vi "Intersperse Data with Invalid Data (single channel).vi"(7 "Intersperse Ratio":dbl=0.1, 10 "Input Data":dbl[](array[numeric]) format="%.16g") -> (1 "Data Valid":bool[](array[boolean]), 2 "Output Data":dbl[](array[numeric]))   [LabVIEW 2011]
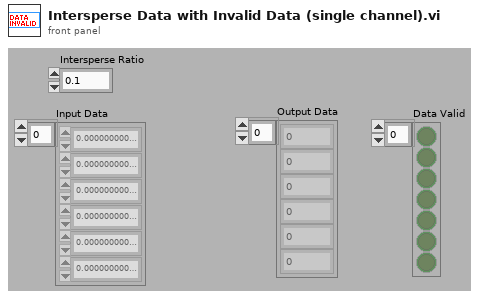
[diagram p1: front panel]
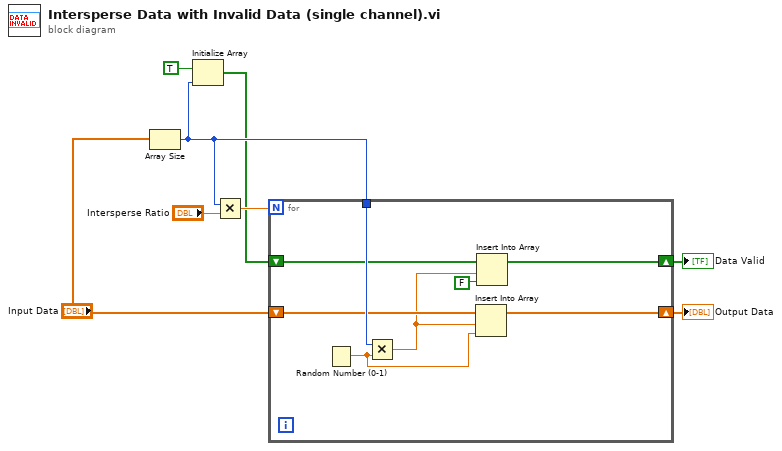
[diagram p0: block diagram]
diagram:
  n1 = Array Size(array="Input Data") -> (size(s)=w5:i32)
  n2 = Initialize Array(TRUE, w5) -> (w3:bool[])
  n3 = Multiply(x=w5, y="Intersperse Ratio") -> (x*y=w8:dbl)
  n4 = for {
    N: w8 -> [_]
    tunnel: w5 -> [w16]
    shift-right: [w13] -> w1
    shift-left: "Input Data" -> [w15]
    shift-right: [w11] -> w2
    shift-left: w3 -> [w12]
    n5 = Random Number (0-1)() -> (number: 0 to 1=w14:dbl)
    n6 = Multiply(x=w16, y=w14) -> (x*y=w10:dbl)
    n7 = Insert Into Array(array=w15, index=w10, new element=w14) -> (w13:dbl[])
    n8 = Insert Into Array(array=w12, index=w10, new element=FALSE) -> (w11:bool[])
  }
  "Data Valid" <- w2
  "Output Data" <- w1
